vi "Update Active Routes.vi"(8 "error in":errorcluster, 11 "2525 in":refnum<class "2525.lvclass">) -> (0 "error out":errorcluster, 3 "2525 out":refnum<class "2525.lvclass">)   [LabVIEW 2019, in "2525.lvlib" / "2525.lvclass"]
uses:
  Library/2525.lvclass
  Library/2525.lvclass/2525.ctl
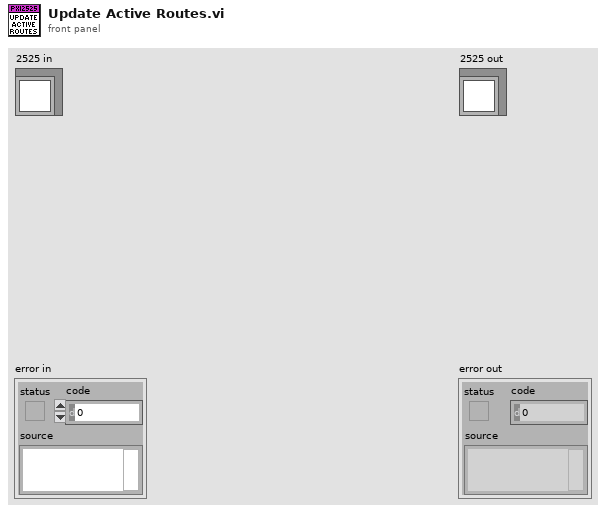
[diagram p1: front panel]
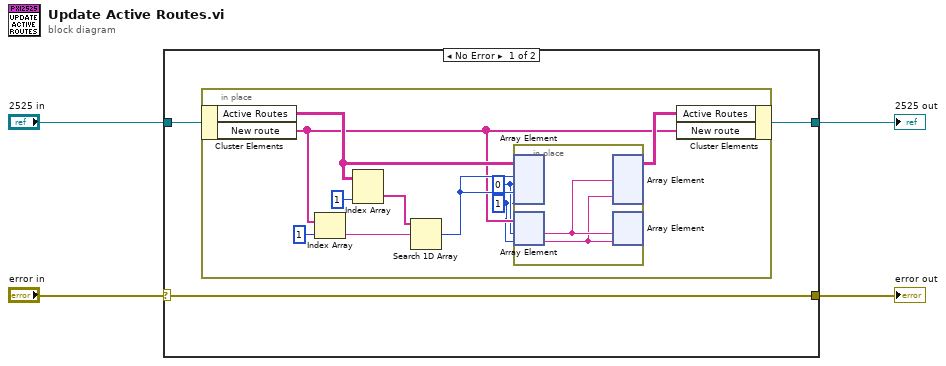
[diagram p0: block diagram]
diagram:
  n1 = case shown="No Error" "error in" {
    selector: "error in" -> [w5 w21]
    tunnel: "2525 in" -> [w7 w20]
    tunnel: [w6 w20] -> w3
    tunnel: [w5 w21] -> w1
    frame No Error {
      n2 = in-place {
        w8 = 1
        w9 = 0
        n3 = in-place-cluster #1(w7) -> ("Active Routes"=w13:string[][], "New route"=w10:string[])
        n4 = Index Array(array=w10, index=1) -> (element=w16:string)
        n5 = Index Array(array=w13, index (col)=1 ("disabled index (col)")) -> (element=w17:string[])  [unwired: 1 in]
        n6 = Search 1D Array(1D array=w17, element=w16) -> (index of element=w11:i32)  [unwired: 1 in]
        n7 = in-place {
          n8 = in-place-array #2(w13, w11, w9, w11, w8) -> ()  [unwired: 2 out]
          n9 = in-place-array #3(w10, w9, w8) -> (w19:string, w18:string)
          n10 = in-place-array #2(w19, w18) -> (w12:string[][])  [unwired: 4 out]
          n11 = in-place-array #3(w19, w18) -> ()  [unwired: 3 out]
        }
        n12 = in-place-cluster #1("Active Routes"=w12, "New route"=w10) -> (w6:refnum<class "2525.lvclass">)
      }
    }
    frame Error {
    }
  }
  "error out" <- w1
  "2525 out" <- w3
